vi "Pack Kalman Data.vi"(10 "output valid":bool, 11 "Data":u16) -> (2 "output valid?":bool, 3 "packer out":T1)   [LabVIEW 2015]
uses:
  OpenScan Labview code_20170126/DRAM data index.ctl
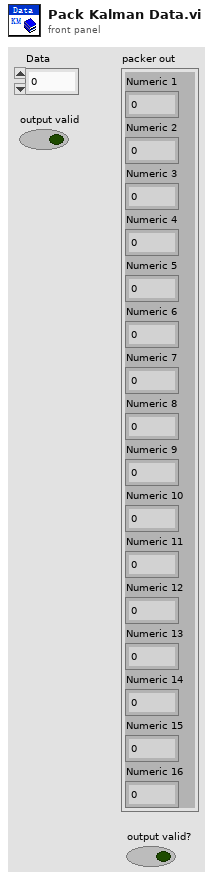
[diagram p1: front panel]
types:
  T1 = cluster{"Numeric 1":u32, "Numeric 2":u32, "Numeric 3":u32, "Numeric 4":u32, "Numeric 5":u32, "Numeric 6":u32, "Numeric 7":u32, "Numeric 8":u32, "Numeric 9":u32, "Numeric 10":u32, "Numeric 11":u32, "Numeric 12":u32, "Numeric 13":u32, "Numeric 14":u32, "Numeric 15":u32, "Numeric 16":u32}
  T2 = typedef "DRAM data index.ctl" = enum16{"Numeric 1", "Numeric 2", "Numeric 3", "Numeric 4", "Numeric 5", "Numeric 6", "Numeric 7", "Numeric 8", "Numeric 9", "Numeric 10", "Numeric 11", "Numeric 12", "Numeric 13", "Numeric 14", "Numeric 15", "Numeric 16"}
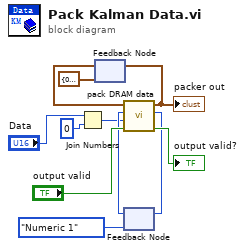
[diagram p0: block diagram]
diagram:
  n1 = Join Numbers(hi="Data", lo=u16 0) -> ((hi.lo)=w1:u32)
  n2 = feedback #1(T1 {"Numeric 1"=0, "Numeric 2"=0, "Numeric 3"=0, "Numeric 4"=0, "Numeric 5"=0, "Numeric 6"=0, "Numeric 7"=0, "Numeric 8"=0, "Numeric 9"=0, "Numeric 10"=0, "Numeric 11"=0, "Numeric 12"=0, "Numeric 13"=0, "Numeric 14"=0, "Numeric 15"=0, "Numeric 16"=0} ("packer out")) -> (w8:T1)
  n3 = feedback #2(DRAM_data_index."Numeric 1" ("DRAM Index out")) -> (w5:T2)
  n4 = call "pack DRAM data.vi"("input valid?"="output valid", "data to be packed"=w1, "DRAM Index in"=w5, "packer in"=w8) -> ("output valid?"=→"output valid?":bool, "DRAM Index out"=w4:T2, "packer out"=w9:T1)  [unwired: 5 in]
  "packer out" <- w9
  n5 = feedback-in #1(w9) -> ()
  n6 = feedback-in #2(w4) -> ()
